vi "tm_setpropertyvalue.vi"(8 "error in (no error)":errorcluster, 9 "Value in":sgl, 10 "Property ID":u32, 11 "Handle in":u32) -> (0 "error out":errorcluster, 3 "Handle out":u32)   [LabVIEW 2016]
uses:
  tmcamcon.dll
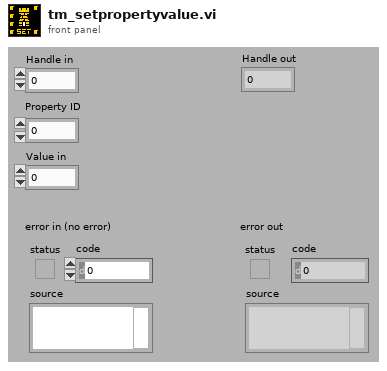
[diagram p1: front panel]
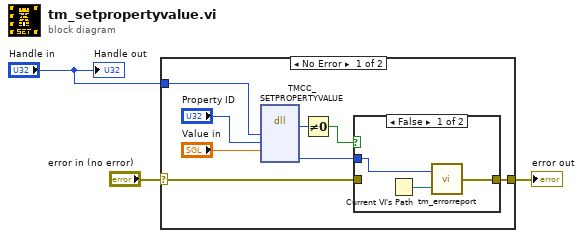
[diagram p0: block diagram]
diagram:
  n1 = case shown="No Error" "error in (no error)" {
    selector: "error in (no error)" -> [w8 w16]
    tunnel: [w5 w16] -> w2
    tunnel: "Handle in" -> [w4 _]
    frame No Error {
      n2 = dll-call lib="tmcamcon.dll" fn="TMCC_SETPROPERTYVALUE"("HDCAM"=w4, "propertyid"="Property ID", "value"="Value in") -> ("return type"=w11:u32, "Erval"=w7:i32)  [unwired: 7 in, 2 out]
      n3 = Not Equal To 0?(x=w11) -> (x != 0?=w6:bool)
      n4 = case shown="False" w6 {
        tunnel: w8 -> [_ w15]
        tunnel: [w13 w15] -> w5
        tunnel: w7 -> [w12 _]
        frame False {
          n5 = Current VI's Path() -> (path=w14:path)
          n6 = call <userlib>:"tm_errorreport.vi"("Source"=w14, "Error"=w12) -> ("error out"=w13:errorcluster)
        }
        frame True {
        }
      }
    }
    frame Error {
    }
  }
  "error out" <- w2
  "Handle out" <- "Handle in"
